vi "UTM na współrzędne dziesiętne.vi"(6 "Parametry Ziemi":T3={"a - półoś duża"=6378137.0, "b - półoś mała"=6356752.3141999999998} {"b - półoś mała" format="%_20f"; "a - półoś duża" format="%_20g"}, 9 "UTM":T2={"E_coord[m]"=393271.81, "N_coord[m]"=5734673.27, "Strefa"=""} {"N_coord[m]" format="%.8g"}) -> (2 "Położenie we współrzędnych geograficznych":T1 {"lambda - długość geograficzna" format="%.20g"; "fi - szerokość geograficzna" format="%.20g"})   [LabVIEW 2015, in "Biblioteka moduł map v3.lvlib" / "Konwersja wsp.lvlib" / "UTM.lvlib"]
doc: "Zadaniem pliku jest wyznaczenie długości i szerokości geograficznej na podstawie pozycji UTM oraz parametrów odwzorowania Ziemi."
uses:
  UTM.lvlib
  <vilib>/regexp/Match Regular Expression.xnode
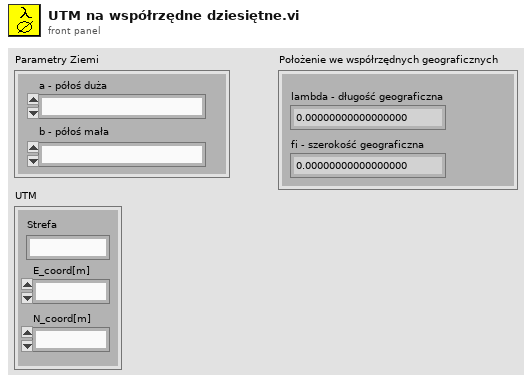
[diagram p1: front panel]
types:
  T1 = cluster{"fi - szerokość geograficzna":ext, "lambda - długość geograficzna":ext}
  T2 = cluster{"E_coord[m]":ext, "N_coord[m]":ext, "Strefa":string}
  T3 = cluster{"a - półoś duża":ext, "b - półoś mała":ext}
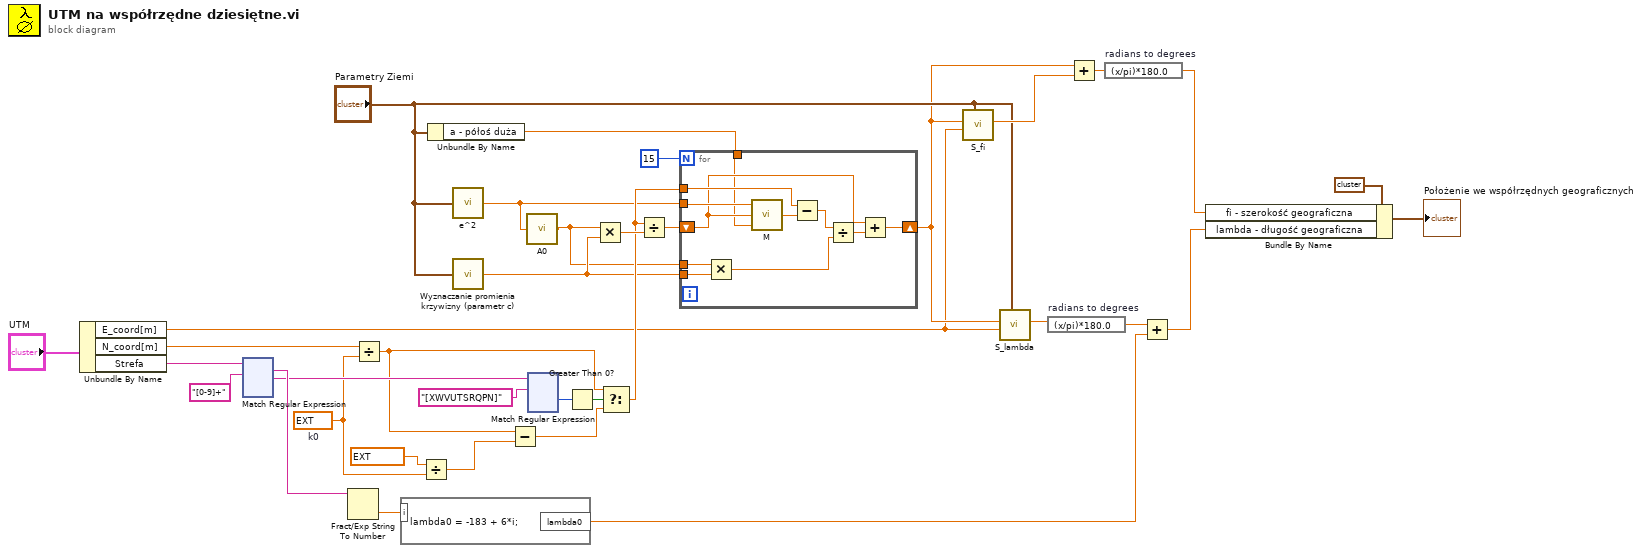
[diagram p0: block diagram]
diagram:
  w17 = ext 0.9996  # k0
  n1 = Unbundle By Name("UTM") -> ("E_coord[m]"=w1:ext, "N_coord[m]"=w9:ext, "Strefa"=w8:string)
  n2 = xnode "Match Regular Expression"("input string"=w8, "regular expression"="[0-9]+") -> ("whole match"=w27:string, "after match"=w25:string)  [unwired: 4 in, 3 out]
  n3 = Fract/Exp String To Number(string=w27) -> (number=w34:dbl)  [unwired: 3 in, 1 out]
  n4 = Divide(x=w9, y=w17) -> (x/y=w21:ext)
  n5 = formula code="lambda0 = -183 + 6*i;"("i"=w34) -> ("lambda0"=w29:dbl)
  n6 = Divide(x=ext 10000000.0 ("y"), y=w17) -> (x/y=w19:ext)
  n7 = Unbundle By Name("Parametry Ziemi") -> ("a - półoś duża"=w16:ext)
  n8 = call "e^2.vi"("Parametry Ziemi"="Parametry Ziemi") -> ("e^2"=w7:ext)  [unwired: 4 in]
  n9 = call "Wyznaczanie promienia krzywizny (parametr c).vi"("Parametry Ziemi"="Parametry Ziemi") -> ("c- promień krzywizny"=w15:ext)  [unwired: 4 in]
  n10 = Subtract(x=w21, y=w19) -> (x-y=w23:ext)
  n11 = call "A0.vi"("e^2"=w7) -> ("A0"=w6:ext)  [unwired: 4 in]
  n12 = xnode "Match Regular Expression"("input string"=w25, "regular expression"="[XWVUTSRQPN]") -> ("offset past match"=w24:i32)  [unwired: 4 in, 4 out]
  n13 = Greater Than 0?(x=w24) -> (x > 0?=w22:bool)
  n14 = Multiply(x=w6, y=w15) -> (x*y=w31:ext)
  n15 = Select(t=w21, s=w22, f=w23) -> (s? t:f=w20:ext)
  n16 = Divide(x=w20, y=w31) -> (x/y=w32:ext)
  n17 = for {
    N: 15 -> [_]
    shift-right: [w42] -> w3
    shift-left: w32 -> [w37]
    tunnel: w20 -> [w44]
    tunnel: w15 -> [w41]
    tunnel: w16 -> [w36]
    tunnel: w7 -> [w38]
    tunnel: w6 -> [w40]
    n18 = Multiply(x=w40, y=w41) -> (x*y=w45:ext)
    n19 = call "M.vi"("a"=w36, "fi[rad]"=w37, "e^2"=w38) -> ("M"=w39:ext)
    n20 = Subtract(x=w44, y=w39) -> (x-y=w43:ext)
    n21 = Divide(x=w43, y=w45) -> (x/y=w46:ext)
    n22 = Add(x=w37, y=w46) -> (x+y=w42:ext)
  }
  n23 = call "S_fi.vi"("Parametry Ziemi"="Parametry Ziemi", "E"=w1, "fi'"=w3) -> ("S_fi"=w5:ext)  [unwired: 7 in]
  n24 = call "S_lambda.vi"("Parametry Ziemi"="Parametry Ziemi", "E"=w1, "fi'[stopnie]"=w3) -> ("S_lambda"=w2:ext)  [unwired: 7 in]
  n25 = expression code="(x/pi)*180.0" "radians to degrees"(w2) -> (w30:ext)
  n26 = Add(x=w3, y=w5) -> (x+y=w28:ext)
  n27 = expression code="(x/pi)*180.0" "radians to degrees"(w28) -> (w11:ext)
  n28 = Add(x=w30, y=w29) -> (x+y=w12:ext)
  n29 = Bundle By Name(cluster=T1 {"fi - szerokość geograficzna"=0.0, "lambda - długość geograficzna"=0.0} ("Położenie we współrzędnych geograficznych 2"), "fi - szerokość geograficzna"=w11, "lambda - długość geograficzna"=w12) -> (→"Położenie we współrzędnych geograficznych":T1)
